vi "ConvertDiagPacket.vi"(8 "error in (no error)":errorcluster, 9 "axisMask":i32, 10 "diagPacket":refnum<k24>, 11 "controller in":refnum<k24>) -> (0 "error out":errorcluster, 2 "LabVIEW data out":T2, 3 "controller out":refnum<k24>)   [LabVIEW 2020]
uses:
  ControllerDiagPacket.ctl
  AxisDiagPacket.ctl
  C:/Program Files (x86)/Aerotech/A3200/LabVIEW/2010/Bin/Aerotech.A3200.dll
  Program Files (x86)/Aerotech/A3200/LabVIEW/2010/Bin/Aerotech.A3200.dll
  C:/Program Files (x86)/Aerotech/A3200/LabVIEW/2010/Bin/Aerotech.A3200.LabVIEW.dll
  Program Files (x86)/Aerotech/A3200/LabVIEW/2010/Bin/Aerotech.A3200.LabVIEW.dll
panel:
  in  "AxisDiagPacket Type 2":T1
  in  "ControllerDiagPacket Type":T2
  in  "AxisDiagPacket Type":T1
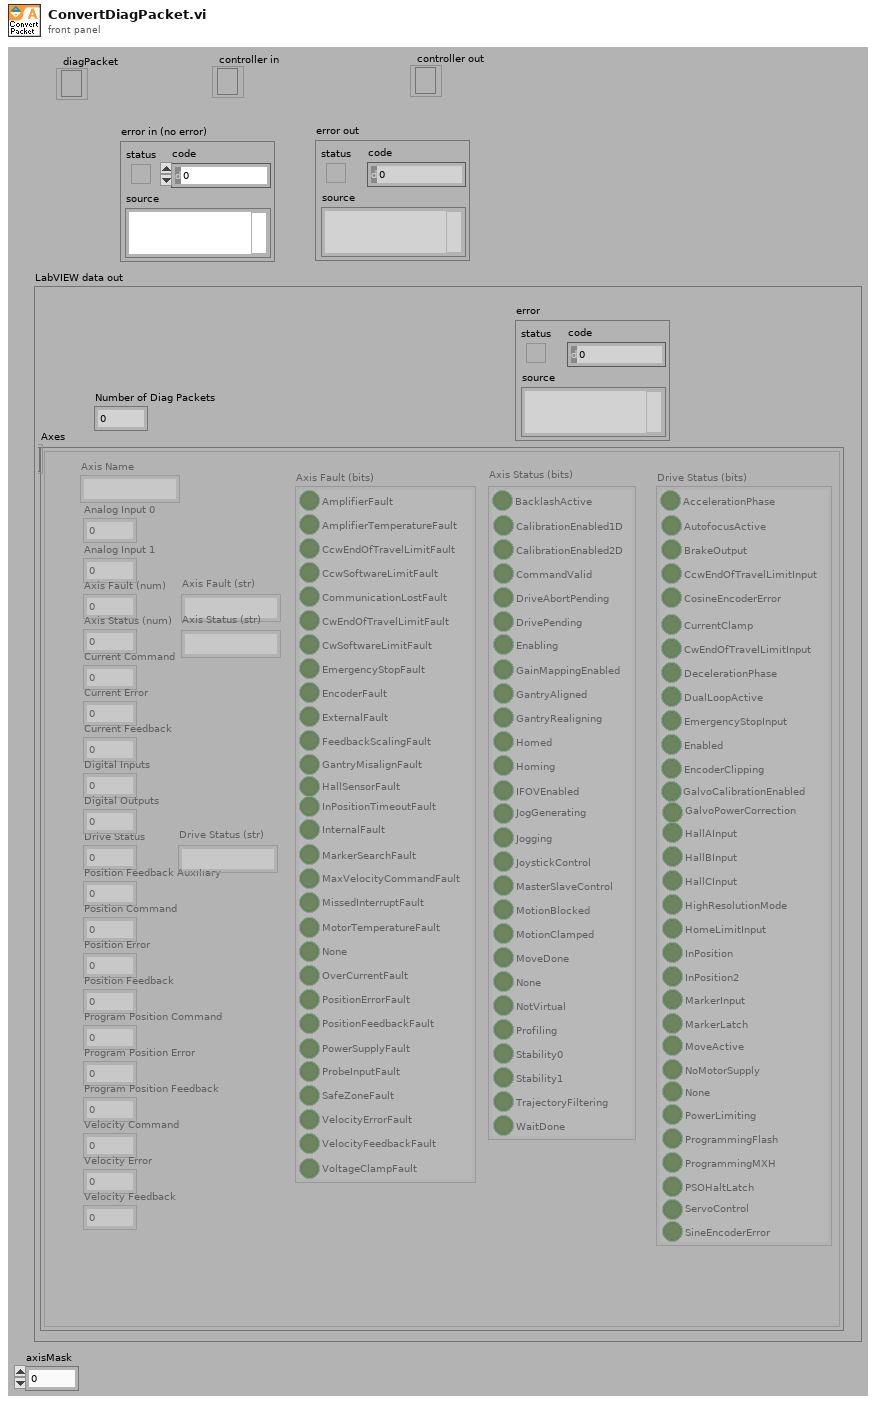
[diagram p1: front panel]
types:
  T1 = typedef "AxisDiagPacket.ctl" = cluster{"Axis Name":string, "Analog Input 0":dbl, "Analog Input 1":dbl, "Axis Fault (num)":i32, "Axis Fault (str)":string, "Axis Fault (bits)":cluster{"AmplifierFault":bool, "AmplifierTemperatureFault":bool, "CcwEndOfTravelLimitFault":bool, "CcwSoftwareLimitFault":bool, "CommunicationLostFault":bool, "CwEndOfTravelLimitFault":bool, "CwSoftwareLimitFault":bool, "EmergencyStopFault":bool, "EncoderFault":bool, "ExternalFault":bool, "FeedbackScalingFault":bool, "GantryMisalignFault ":bool, "HallSensorFault":bool, "InPositionTimeoutFault":bool, "InternalFault":bool, "MarkerSearchFault":bool, "MaxVelocityCommandFault":bool, "MissedInterruptFault":bool, "MotorTemperatureFault":bool, "None":bool, "OverCurrentFault":bool, "PositionErrorFault":bool, "PositionFeedbackFault":bool, "PowerSupplyFault":bool, "ProbeInputFault":bool, "SafeZoneFault":bool, "VelocityErrorFault":bool, "VelocityFeedbackFault":bool, "VoltageClampFault":bool}, "Axis Status (num)":i32, "Axis Status (str)":string, "Axis Status (bits)":cluster{"BacklashActive":bool, "CalibrationEnabled1D":bool, "CalibrationEnabled2D":bool, "CommandValid":bool, "DriveAbortPending":bool, "DrivePending":bool, "Enabling":bool, "GainMappingEnabled":bool, "GantryAligned":bool, "GantryRealigning":bool, "Homed":bool, "Homing":bool, "IFOVEnabled":bool, "JogGenerating":bool, "Jogging":bool, "JoystickControl":bool, "MasterSlaveControl":bool, "MotionBlocked":bool, "MotionClamped":bool, "MoveDone":bool, "None":bool, "NotVirtual":bool, "Profiling":bool, "Stability0":bool, "Stability1":bool, "TrajectoryFiltering":bool, "WaitDone":bool}, "Current Command":sgl, "Current Error":sgl, "Current Feedback":sgl, "Digital Inputs":i32, "Digital Outputs":i32, "Drive Status":i32, "Drive Status (str)":string, "Drive Status (bits)":cluster{"AccelerationPhase":bool, "AutofocusActive":bool, "BrakeOutput":bool, "CcwEndOfTravelLimitInput":bool, "CosineEncoderError":bool, "CurrentClamp":bool, "CwEndOfTravelLimitInput":bool, "DecelerationPhase":bool, "DualLoopActive":bool, "EmergencyStopInput":bool, "Enabled":bool, "EncoderClipping":bool, "GalvoCalibrationEnabled":bool, "GalvoPowerCorrection":bool, "HallAInput":bool, "HallBInput":bool, "HallCInput":bool, "HighResolutionMode":bool, "HomeLimitInput":bool, "InPosition":bool, "InPosition2":bool, "MarkerInput":bool, "MarkerLatch":bool, "MoveActive":bool, "NoMotorSupply":bool, "None":bool, "PowerLimiting":bool, "ProgrammingFlash":bool, "ProgrammingMXH":bool, "PSOHaltLatch":bool, "ServoControl":bool, "SineEncoderError":bool}, "Position Feedback Auxiliary":dbl, "Position Command":dbl, "Position Error":dbl, "Position Feedback":dbl, "Program Position Command":dbl, "Program Position Error":dbl, "Program Position Feedback":dbl, "Velocity Command":dbl, "Velocity Error":dbl, "Velocity Feedback":dbl}
  T2 = typedef "ControllerDiagPacket.ctl" = cluster{"Number of Diag Packets":i32, "Axes":T1[], "error":errorcluster}
  T3 = cluster{dbl, dbl, dbl, dbl, dbl, dbl, dbl, dbl, dbl, dbl}
  T4 = cluster{"driveStatusBits[0]":bool, "driveStatusBits[1]":bool, "driveStatusBits[2]":bool, "driveStatusBits[3]":bool, "driveStatusBits[4]":bool, "driveStatusBits[5]":bool, "driveStatusBits[6]":bool, "driveStatusBits[7]":bool, "driveStatusBits[8]":bool, "driveStatusBits[9]":bool, "driveStatusBits[10]":bool, "driveStatusBits[11]":bool, "driveStatusBits[12]":bool, "driveStatusBits[13]":bool, "driveStatusBits[14]":bool, "driveStatusBits[15]":bool, "driveStatusBits[16]":bool, "driveStatusBits[17]":bool, "driveStatusBits[18]":bool, "driveStatusBits[19]":bool, "driveStatusBits[20]":bool, "driveStatusBits[21]":bool, "driveStatusBits[22]":bool, "driveStatusBits[23]":bool, "driveStatusBits[24]":bool, "driveStatusBits[25]":bool, "driveStatusBits[26]":bool, "driveStatusBits[27]":bool, "driveStatusBits[28]":bool, "driveStatusBits[29]":bool, "driveStatusBits[30]":bool, "driveStatusBits[31]":bool}
  T5 = cluster{"axisStatusBits[0]":bool, "axisStatusBits[1]":bool, "axisStatusBits[2]":bool, "axisStatusBits[3]":bool, "axisStatusBits[4]":bool, "axisStatusBits[5]":bool, "axisStatusBits[6]":bool, "axisStatusBits[7]":bool, "axisStatusBits[8]":bool, "axisStatusBits[9]":bool, "axisStatusBits[10]":bool, "axisStatusBits[11]":bool, "axisStatusBits[12]":bool, "axisStatusBits[13]":bool, "axisStatusBits[14]":bool, "axisStatusBits[15]":bool, "axisStatusBits[16]":bool, "axisStatusBits[17]":bool, "axisStatusBits[18]":bool, "axisStatusBits[19]":bool, "axisStatusBits[20]":bool, "axisStatusBits[21]":bool, "axisStatusBits[22]":bool, "axisStatusBits[23]":bool, "axisStatusBits[24]":bool, "axisStatusBits[25]":bool, "axisStatusBits[26]":bool}
  T6 = cluster{"axisFaultBits[0]":bool, "axisFaultBits[1]":bool, "axisFaultBits[2]":bool, "axisFaultBits[3]":bool, "axisFaultBits[4]":bool, "axisFaultBits[5]":bool, "axisFaultBits[6]":bool, "axisFaultBits[7]":bool, "axisFaultBits[8]":bool, "axisFaultBits[9]":bool, "axisFaultBits[10]":bool, "axisFaultBits[11]":bool, "axisFaultBits[12]":bool, "axisFaultBits[13]":bool, "axisFaultBits[14]":bool, "axisFaultBits[15]":bool, "axisFaultBits[16]":bool, "axisFaultBits[17]":bool, "axisFaultBits[18]":bool, "axisFaultBits[19]":bool, "axisFaultBits[20]":bool, "axisFaultBits[21]":bool, "axisFaultBits[22]":bool, "axisFaultBits[23]":bool, "axisFaultBits[24]":bool, "axisFaultBits[25]":bool, "axisFaultBits[26]":bool, "axisFaultBits[27]":bool, "axisFaultBits[28]":bool}
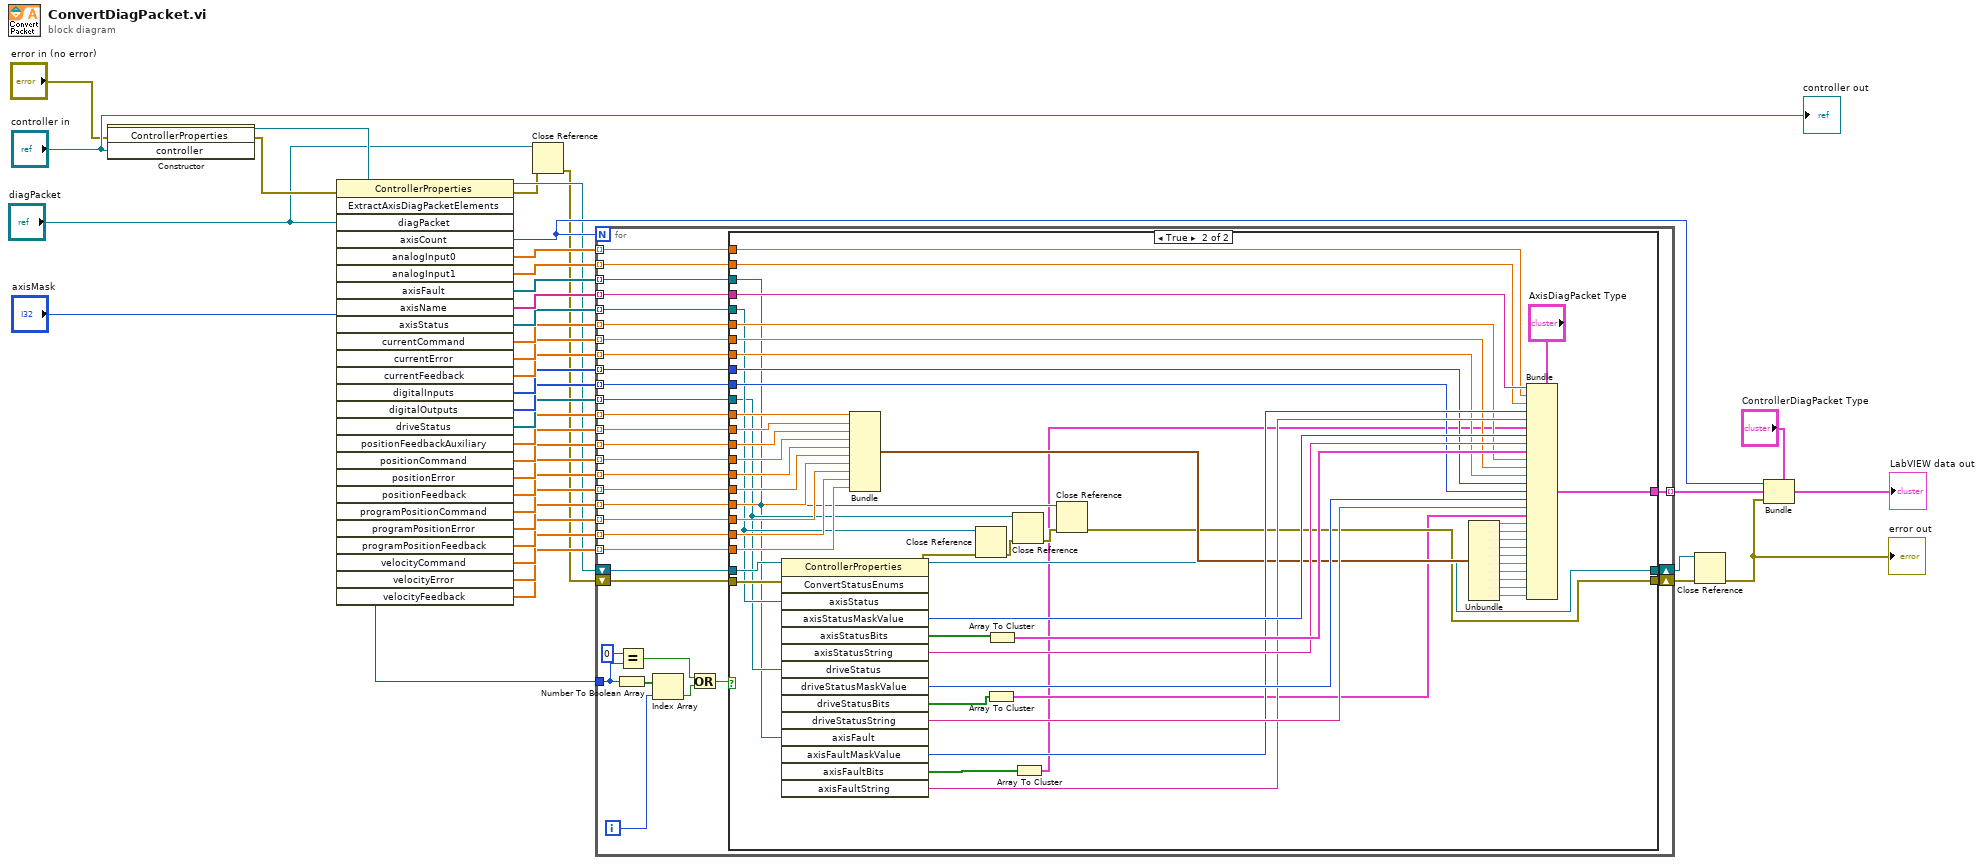
[diagram p0: block diagram]
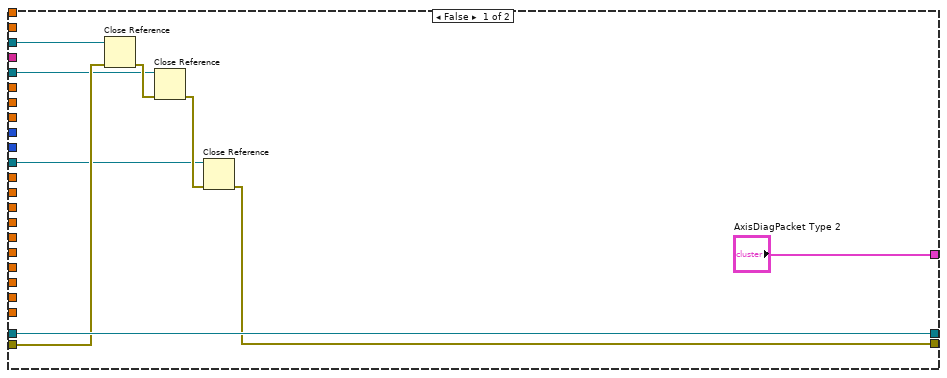
[diagram p2: hidden frame]
diagram:
  n1 = constructor class="ControllerProperties"(error in="error in (no error)", "controller"="controller in") -> (reference out=w35:refnum<k24>, error out=w9:errorcluster)  [unwired: 2 in, 2 out]
  n2 = invoke class="ControllerProperties" method="ExtractAxisDiagPacketElements"(reference=w35, error in=w9, "diagPacket"="diagPacket") -> (reference out=w8:refnum<k24>, error out=w3:errorcluster, "axisCount"=w11:i32, "analogInput0"=w34:dbl[], "analogInput1"=w33:dbl[], "axisFault"=w32:refnum<k24>[], "axisName"=w31:string[], "axisStatus"=w30:refnum<k24>[], "currentCommand"=w29:sgl[], "currentError"=w28:sgl[], "currentFeedback"=w27:sgl[], "digitalInputs"=w26:i32[], "digitalOutputs"=w25:i32[], "driveStatus"=w24:refnum<k24>[], "positionFeedbackAuxiliary"=w23:dbl[], "positionCommand"=w22:dbl[], "positionError"=w21:dbl[], "positionFeedback"=w20:dbl[], "programPositionCommand"=w19:dbl[], "programPositionError"=w18:dbl[], "programPositionFeedback"=w17:dbl[], "velocityCommand"=w16:dbl[], "velocityError"=w15:dbl[], "velocityFeedback"=w14:dbl[])  [unwired: 23 in, 2 out]
  n3 = Close Reference(reference="diagPacket", error in (no error)=w3) -> (error out=w2:errorcluster)
  n4 = for {
    N: w11 -> [_]
    tunnel: w34 -> [w66] mode=indexing
    tunnel: w33 -> [w65] mode=indexing
    tunnel: w32 -> [w67] mode=indexing
    tunnel: w31 -> [w70] mode=indexing
    tunnel: w30 -> [w69] mode=indexing
    tunnel: w29 -> [w64] mode=indexing
    tunnel: w28 -> [w63] mode=indexing
    tunnel: w27 -> [w62] mode=indexing
    tunnel: w26 -> [w61] mode=indexing
    tunnel: w25 -> [w60] mode=indexing
    tunnel: w24 -> [w68] mode=indexing
    tunnel: w23 -> [w59] mode=indexing
    tunnel: w22 -> [w58] mode=indexing
    tunnel: w21 -> [w57] mode=indexing
    tunnel: w20 -> [w56] mode=indexing
    tunnel: w19 -> [w55] mode=indexing
    tunnel: w18 -> [w54] mode=indexing
    tunnel: w17 -> [w53] mode=indexing
    tunnel: w16 -> [w52] mode=indexing
    tunnel: w15 -> [w51] mode=indexing
    tunnel: w14 -> [w50] mode=indexing
    tunnel: [w49] -> w12 mode=indexing
    shift-right: [w46] -> w7
    shift-left: w8 -> [w48]
    shift-right: [w45] -> w6
    shift-left: w2 -> [w47]
    tunnel: "axisMask" -> [w44]
    i -> [w41]
    n5 = Number To Boolean Array(number=w44) -> (Boolean array=w42:bool[])
    n6 = Equal?(x=0, y=w44) -> (x = y?=w38:bool)
    n7 = Index Array(array=w42, index=w41) -> (element=w39:bool)
    n8 = Or(x=w38, y=w39) -> (x .or. y?=w40:bool)
    n9 = case shown="True" w40 {
      tunnel: w70 -> [_ w131]
      tunnel: w69 -> [w74 w88]
      tunnel: w68 -> [w72 w84]
      tunnel: w67 -> [w76 w83]
      tunnel: w66 -> [_ w122]
      tunnel: w65 -> [_ w121]
      tunnel: w64 -> [_ w120]
      tunnel: w63 -> [_ w119]
      tunnel: w62 -> [_ w118]
      tunnel: w61 -> [_ w117]
      tunnel: w60 -> [_ w116]
      tunnel: w59 -> [_ w115]
      tunnel: w58 -> [_ w114]
      tunnel: w57 -> [_ w113]
      tunnel: w56 -> [_ w112]
      tunnel: w55 -> [_ w111]
      tunnel: w54 -> [_ w110]
      tunnel: w53 -> [_ w109]
      tunnel: w52 -> [_ w108]
      tunnel: w51 -> [_ w107]
      tunnel: w50 -> [_ w106]
      tunnel: ["AxisDiagPacket Type 2" w94] -> w49
      tunnel: w48 -> [w78 w93]
      tunnel: w47 -> [w77 w92]
      tunnel: [w78 w91] -> w46
      tunnel: [w71 w85] -> w45
      frame False {
        n10 = Close Reference(reference=w76, error in (no error)=w77) -> (error out=w75:errorcluster)
        n11 = Close Reference(reference=w74, error in (no error)=w75) -> (error out=w73:errorcluster)
        n12 = Close Reference(reference=w72, error in (no error)=w73) -> (error out=w71:errorcluster)
      }
      frame True {
        n13 = invoke class="ControllerProperties" method="ConvertStatusEnums"(reference=w93, error in=w92, "axisStatus"=w88, "driveStatus"=w84, "axisFault"=w83) -> (reference out=w91:refnum<k24>, error out=w89:errorcluster, "axisStatusMaskValue"=w128:i32, "axisStatusBits"=w130:bool[], "axisStatusString"=w127:string, "driveStatusMaskValue"=w126:i32, "driveStatusBits"=w81:bool[], "driveStatusString"=w125:string, "axisFaultMaskValue"=w124:i32, "axisFaultBits"=w90:bool[], "axisFaultString"=w123:string)  [unwired: 10 in, 4 out]
        n14 = Bundle(w115, w114, w113, w112, w111, w110, w109, w108, w107, w106) -> (w105:T3)  [unwired: 1 in]
        n15 = Close Reference(reference=w88, error in (no error)=w89) -> (error out=w87:errorcluster)
        n16 = Array To Cluster(array=w81) -> (cluster=w82:T4)
        n17 = Array To Cluster(array=w130) -> (cluster=w129:T5)
        n18 = Close Reference(reference=w84, error in (no error)=w87) -> (error out=w86:errorcluster)
        n19 = Array To Cluster(array=w90) -> (cluster=w80:T6)
        n20 = Close Reference(reference=w83, error in (no error)=w86) -> (error out=w85:errorcluster)
        n21 = Unbundle(w105) -> (w104:dbl, w103:dbl, w102:dbl, w101:dbl, w100:dbl, w99:dbl, w98:dbl, w97:dbl, w96:dbl, w95:dbl)
        n22 = Bundle(cluster="AxisDiagPacket Type", "Axis Name"=w131, "Analog Input 0"=w122, "Analog Input 1"=w121, "Axis Fault (num)"=w124, "Axis Fault (str)"=w123, "Axis Fault (bits)"=w80, "Axis Status (num)"=w128, "Axis Status (str)"=w127, "Axis Status (bits)"=w129, "Current Command"=w120, "Current Error"=w119, "Current Feedback"=w118, "Digital Inputs"=w117, "Digital Outputs"=w116, "Drive Status"=w126, "Drive Status (str)"=w125, "Drive Status (bits)"=w82, "Position Feedback Auxiliary"=w104, "Position Command"=w103, "Position Error"=w102, "Position Feedback"=w101, "Program Position Command"=w100, "Program Position Error"=w99, "Program Position Feedback"=w98, "Velocity Command"=w97, "Velocity Error"=w96, "Velocity Feedback"=w95) -> (w94:T1)
      }
    }
  }
  n23 = Close Reference(reference=w7, error in (no error)=w6) -> (error out=w5:errorcluster)
  "error out" <- w5
  n24 = Bundle(cluster="ControllerDiagPacket Type", "Number of Diag Packets"=w11, "Axes"=w12, "error"=w5) -> (→"LabVIEW data out":T2)
  "controller out" <- "controller in"
